vi "ExCenterStripSpecIN.vi"() -> ()   [LabVIEW 2010]
panel:
  in  "Wavelength":dbl=546.0 format="%.2f"
  in  "Grating Speed":dbl=2000.0 min=1.0 step=1.0 format="%.2f"
  in  "Grating number":i16=1 min=1 max=100 step=1
  out "Strip":sgl[](graph)
  in  "Temperature":dbl=-10.0 format="%.2f"
  in  "Exposure":dbl=0.5 min=0.0 step=0.001 format="%.3f"
  in  "stop":bool
  out "error out":errorcluster
  in  "error in (no error)":errorcluster
  # "ExCenterStripSpecIN.vi (InSpectrum)\nCamera and Spectrometer control of the InSpectrum.  This vi will open both the camera and spectrograph.  It will then move the grating to the Wavelength.  Data will then be collected and displayed until the STOP button is hit."
  # "NOTES:\nA properly configured spectometer .ini must be present in the LabVIEW folder for spectrograph operation.\n\nConsult the Toolkit documentation for more information on how to configure this file."
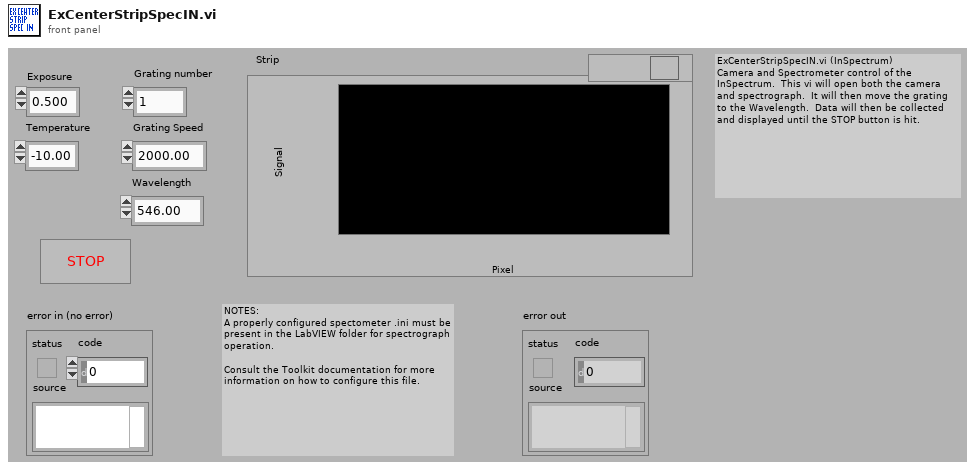
[diagram p1: front panel]
types:
  T1 = cluster{"acquire focus mode":u32, "Exposure":dbl, "Number of Images":u32, "Software accumulation":u32}
  T2 = cluster{"Camera Handle":u32, "Pulser Handle":u32, "File Handle":u32, "Display Handle":u32, "Image Handle":u32}
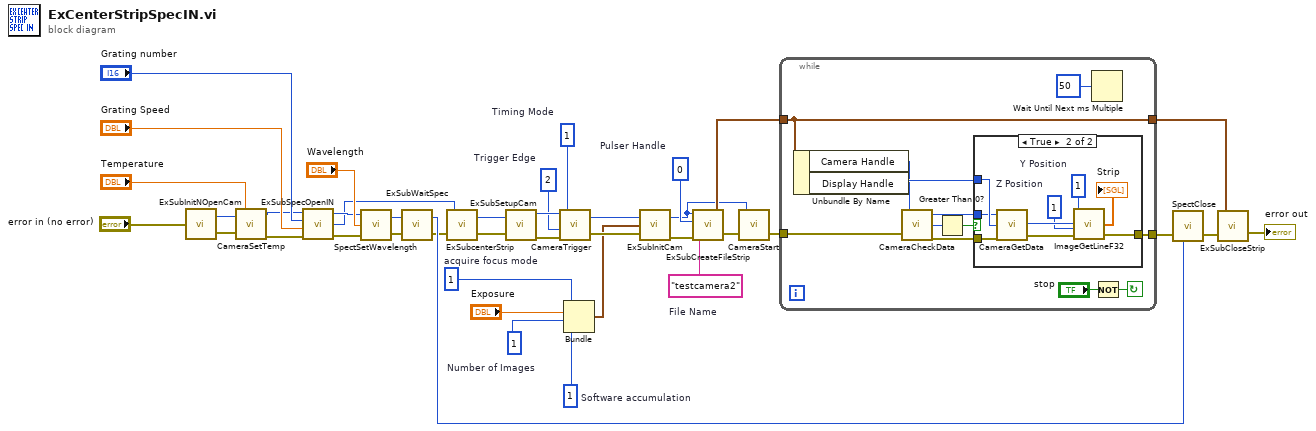
[diagram p0: block diagram]
diagram:
  w15 = u32 0  # Pulser Handle
  w20 = u32 1  # acquire focus mode
  w19 = u32 1  # Number of Images
  w18 = u32 1  # Software accumulation
  w17 = u32 1  # Timing Mode
  w21 = u32 2  # Trigger Edge
  w13 = "testcamera2"  # File Name
  n1 = call "ExSubInitNOpenCam.vi"("error in (no error)"="error in (no error)") -> ("Camera Handle"=w7:u32, "error out"=w6:errorcluster)
  n2 = call <userlib>:"CameraSetTemp.vi"("error in (no error)"=w6, "Temperature"="Temperature", "Camera Handle"=w7) -> ("error out"=w4:errorcluster, "Camera Handle"=w5:u32)
  n3 = call "ExSubSpecOpenIN.vi"("error in (no error)"=w4, "Grating speed"="Grating Speed", "Grating number"="Grating number", "Camera Handles"=w5) -> ("error out"=w26:errorcluster, "Camera Handle"=w11:u32, "Spectrometer Handle"=w25:u32)
  n4 = call <userlib>:"SpectSetWavelength.vi"("error in"=w26, "Wavelength"="Wavelength", "Spectrometer Handle"=w25) -> ("error out"=w28:errorcluster, "Spectrumeter Handle"=w27:u32)
  n5 = call "ExSubWaitSpec.vi"("error in (no error)"=w28, "Spectrometer Handle"=w27) -> ("error out"=w12:errorcluster, "Spectrometer handle"=w23:u32)
  n6 = call "ExSubcenterStrip.vi"("error in (no error)"=w12, "Camera Handle"=w11) -> ("error out"=w1:errorcluster, "Camera Handle"=w2:u32)
  n7 = call "ExSubSetupCam.vi"("error in (no error)"=w1, "Camera Handle"=w2) -> ("error out"=w9:errorcluster, "Camera Handle"=w35:u32)
  n8 = call <userlib>:"CameraTrigger.vi"("error in"=w9, "Trigger Edge"=w21, "Timing Mode"=w17, "Camera Handle"=w35) -> ("error out"=w36:errorcluster, "Camera Handle"=w34:u32)
  n9 = Bundle("acquire focus mode"=w20, "Exposure"="Exposure", "Number of Images"=w19, "Software accumulation"=w18) -> (w16:T1)  [unwired: 1 in]
  n10 = call "ExSubInitCam.vi"("error in (no error)"=w36, "Camera Information"=w16, "Camera Handle"=w34) -> ("error out"=w10:errorcluster, "Camera Handle"=w14:u32)
  n11 = call "ExSubCreateFileStrip.vi"("error in (no error)"=w10, "File and Display Name"=w13, "Pulser Handle"=w15, "Camera Handle"=w14) -> ("error out"=w32:errorcluster, "Handles Out"=w38:T2)
  n12 = call <userlib>:"CameraStart.vi"("error in"=w32, "Camera Handle"=w14) -> ("error out"=w33:errorcluster)  [unwired: 1 out]
  n13 = while {
    tunnel: w38 -> [w49]
    tunnel: w33 -> [w48]
    tunnel: [w46] -> w22
    tunnel: [w49] -> w37
    stop <- w50 continue-if-true
    n14 = Unbundle By Name(w49) -> ("Camera Handle"=w41:u32, "Display Handle"=w45:u32)
    n15 = call <userlib>:"CameraCheckData.vi"("Camera Handle"=w41, "error in"=w48) -> ("Camera Handle"=w42:u32, "Number Of Frames Available"=w43:i32, "error out"=w47:errorcluster)
    n16 = Greater Than 0?(x=w43) -> (x > 0?=w44:bool)
    n17 = case shown="True" w44 {
      tunnel: w47 -> [w53 w61]
      tunnel: [w53 w59] -> w46
      tunnel: w45 -> [_ w57]
      tunnel: w42 -> [_ w56]
      frame False {
      }
      frame True {
        w54 = u32 1  # Z Position
        w55 = u32 1  # Y Position
        n18 = call <userlib>:"CameraGetData.vi"("error in"=w61, "Data Handle"=w57, "Camera Handle"=w56) -> ("error out"=w60:errorcluster, "Data Handle"=w58:u32)  [unwired: 1 out]
        n19 = call <userlib>:"ImageGetLineF32.vi"("error in"=w60, "Z Position"=w54, "Y Position"=w55, "Data Handle"=w58) -> ("error out"=w59:errorcluster, "Array F32"=→"Strip":sgl[])  [unwired: 1 out]
      }
    }
    n20 = Wait Until Next ms Multiple(millisecond multiple=u32 50) -> ()  [unwired: 1 out]
    n21 = Not(x="stop") -> (.not. x?=w50:bool)
  }
  n22 = call <userlib>:"SpectClose.vi"("error in"=w22, "Spectrometer Handle"=w23) -> ("error out"=w24:errorcluster)
  n23 = call "ExSubCloseStrip.vi"("error in (no error)"=w24, "Handles In"=w37) -> ("error out"=→"error out":errorcluster)
